vi "te_configSerial.vi"(2 "Error In":errorcluster, 3 "teSerial":T1={"port"="COM1", "timeout"=4000, "baud"=115200, "dataBits"=8, "stopBits"=10, "flowControl"=0, "parity"=0, "termChar"=FALSE, "checkSum"=FALSE, "checkSumVal"="", "Address"=["01", "02", "03"]} {"stopBits" items=["1.0"=10, "1.5"=15, "2.0"=20]; "flowControl" items=["None"=0, "XON/XOFF"=1, "RTS/CTS"=2, "DTR/DSR"=4]; "parity" items=["None", "Odd", "Even", "Mark", "Space"]}) -> (0 "error out":errorcluster, 1 "VISA resource name out":refnum<visa-resource-name>)   [LabVIEW 2018]
uses:
  TE_Serial_Config_Clust.ctl
  <vilib>/Instr/_visa.llb/VISA Configure Serial Port (Instr).vi
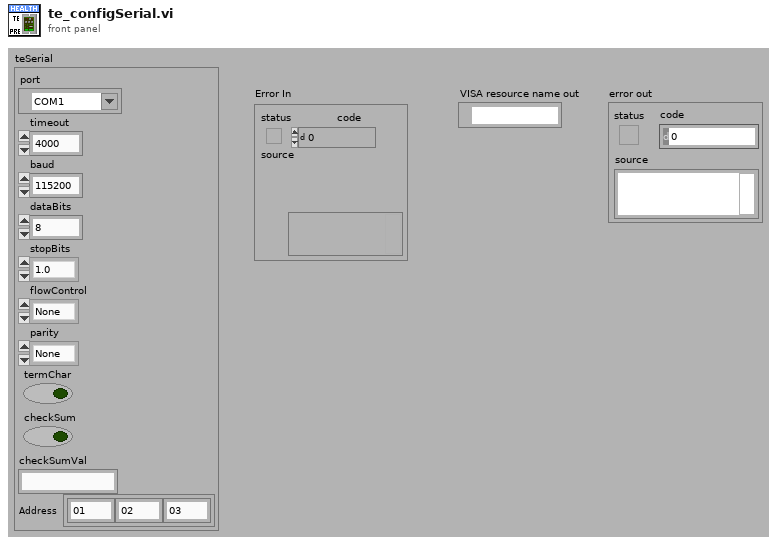
[diagram p1: front panel]
types:
  T1 = typedef "TE_Serial_Config_Clust.ctl" = cluster{"port":refnum<visa-resource-name>, "timeout":u32, "baud":u32, "dataBits":u16, "stopBits":u16, "flowControl":u16, "parity":u16, "termChar":bool, "checkSum":bool, "checkSumVal":string, "Address":string[]}
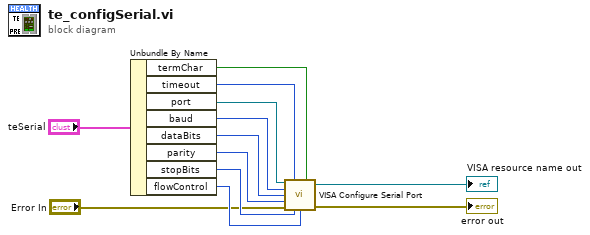
[diagram p0: block diagram]
diagram:
  n1 = Unbundle By Name("teSerial") -> ("termChar"=w5:bool, "timeout"=w6:u32, "port"=w7:refnum<visa-resource-name>, "baud"=w8:u32, "dataBits"=w9:u16, "parity"=w10:u16, "stopBits"=w11:u16, "flowControl"=w12:u16)
  n2 = call-poly "VISA Configure Serial Port"("VISA resource name"=w7, "timeout (10sec)"=w6, "Enable Termination\nChar (T)"=w5, "baud rate (9600)"=w8, "data bits (8)"=w9, "parity (0:none)"=w10, "error in (no error)"="Error In", "stop bits (10: 1 bit)"=w11, "flow control (0:none)"=w12) -> ("VISA resource name out"=→"VISA resource name out":refnum<visa-resource-name>, "error out"=→"error out":errorcluster)  [unwired: 5 in]
